vi "Init.vi"(8 "error in":errorcluster, 10 "Session":string, 11 "Session HVPS in":refnum<class "Session HVPS.lvclass">) -> (0 "error out":errorcluster, 3 "Session HVPS out":refnum<class "Session HVPS.lvclass">)   [LabVIEW 2013, in "Session HVPS.lvclass"]
uses:
  Session HVPS.lvclass
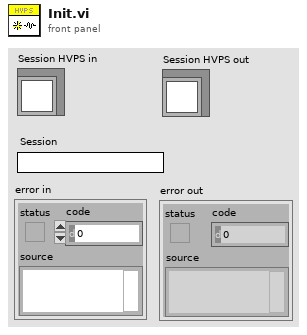
[diagram p1: front panel]
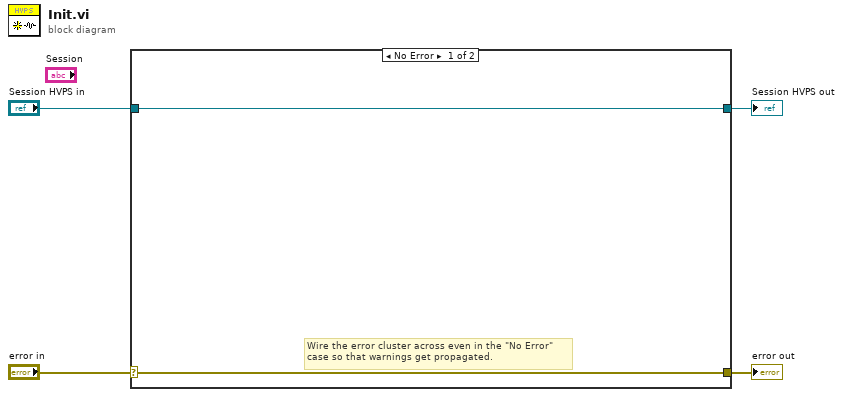
[diagram p0: block diagram]
diagram:
  n1 = case shown="No Error" "error in" {
    selector: "error in" -> [w5 w8]
    tunnel: [w5 w8] -> w3
    tunnel: [w6 w7] -> w1
    tunnel: "Session HVPS in" -> [w6 w7]
    frame No Error {
      # "Wire the error cluster across even in the \"No Error\"\ncase so that warnings get propagated."
    }
    frame Error {
    }
  }
  "error out" <- w3
  "Session HVPS out" <- w1
